vi "write_table_key_string.vi"(7 "table":string="nipm", 8 "error in (no error)":errorcluster, 9 "value":string="6.6.6", 10 "key":string="version", 11 "toml in":refnum<class "toml.lvclass">) -> (0 "error out":errorcluster, 3 "toml out":refnum<class "toml.lvclass">)   [LabVIEW 2020, in "toml.lvclass"]
uses:
  toml.lvclass
  toml.lvclass/toml.ctl
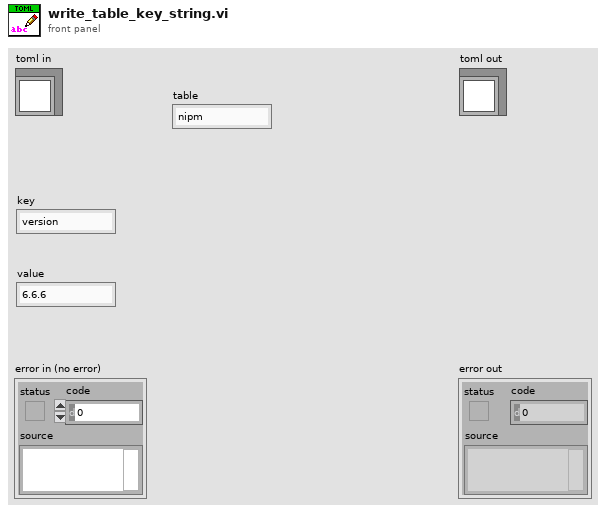
[diagram p1: front panel]
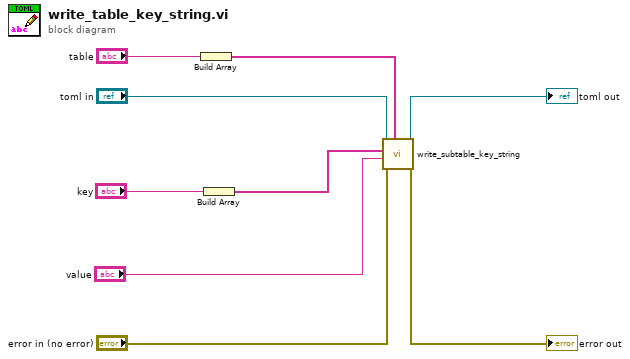
[diagram p0: block diagram]
diagram:
  n1 = Build Array("table") -> (w2:string[])
  n2 = Build Array("key") -> (w1:string[])
  n3 = call "write_subtable_key_string.vi"("subtables"=w2, "error in (no error)"="error in (no error)", "value"="value", "subkeys"=w1, "toml in"="toml in") -> ("error out"=→"error out":errorcluster, "toml out"=→"toml out":refnum<class "toml.lvclass">)  [unwired: 5 in]
